vi "localhost to ip.vi"(11 "hostname":string) -> (3 "true hostname":string)   [LabVIEW 2013, in "TEC editor node.lvclass"]
uses:
  TEC editor node.lvclass
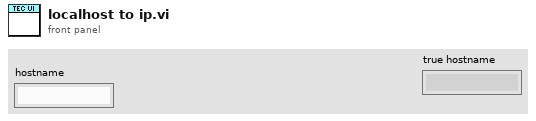
[diagram p1: front panel]
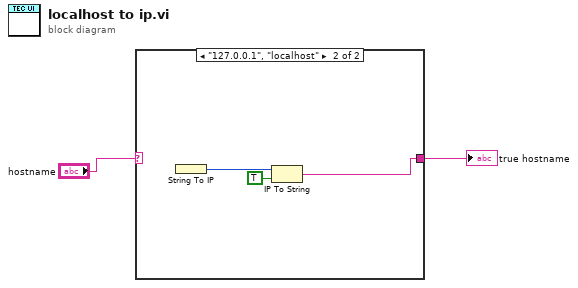
[diagram p0: block diagram]
diagram:
  n1 = case shown="\"127.0.0.1\", \"localhost\"" "hostname" {
    selector: "hostname" -> [w3 _]
    tunnel: [w3 w5] -> w1
    frame Default {
    }
    frame "127.0.0.1", "localhost" {
      n2 = String To IP() -> (0:w6:u32)  [unwired: 1 in]
      n3 = IP To String(1:TRUE ("dot notation? (F)"), 2:w6) -> (0:w5:string)
    }
  }
  "true hostname" <- w1
